vi "initialize.vi"(0 "HGF_FGV_Delete":refnum<class "HGF_FGV_Delete.lvclass">, 3 "initializationData":variant, 5 "error in (no error)":errorcluster, 7 "binaryString":string, 8 "I8 Array":i8[](array[numeric]), 9 "prependSize? (T)":bool, 11 "byteOrder (0:big-endian, network order)":T1(ring)) -> (14 "dup HGF_FGV_Delete":refnum<class "HGF_FGV_Delete.lvclass">, 17 "found?":bool, 19 "error out":errorcluster)   [LabVIEW 2012, in "HGF_FGV.lvlib" / "HGF_FGV_Delete.lvclass"]
doc: "This is a dynamic dispatch VI to be implemented by child classes to initialize their attributes.\n\n<B>Attention:</B> Support for Variant for initialization data only."
uses:
  HGF_FGV_Delete.lvclass
  HGF_FGV_Action/HGF_FGV_Action.lvclass
  HGF_FGV_Delete.lvclass/HGF_FGV_Delete.ctl
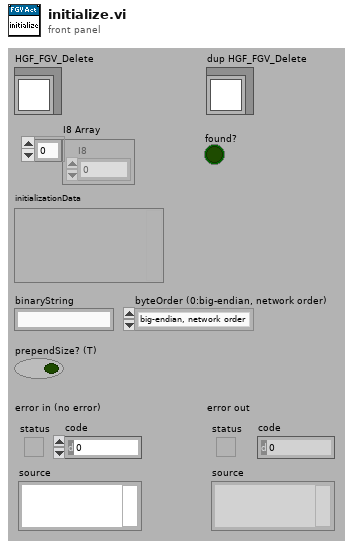
[diagram p1: front panel]
types:
  T1 = enum16{"big-endian, network order", "native, host order", "little-endian"}
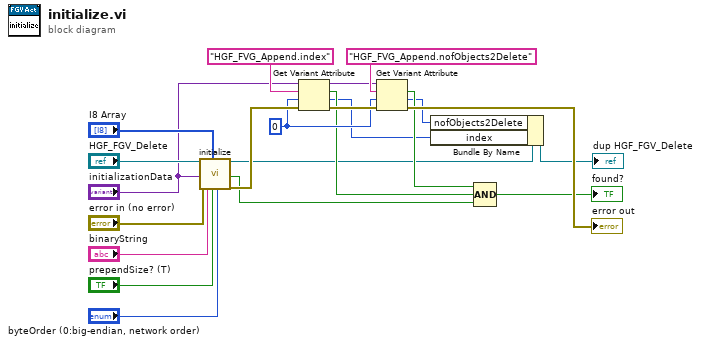
[diagram p0: block diagram]
diagram:
  w14 = u32 0
  n1 = call-parent "initialize.vi"("HGF_Factory"="HGF_FGV_Delete", "initializationData"="initializationData", "error in (no error)"="error in (no error)", "binaryString"="binaryString", "I8 Array"="I8 Array", "prependSize? (T)"="prependSize? (T)", "byteOrder (0:big-endian, network order)"="byteOrder (0:big-endian, network order)") -> ("dup HGF_Factory"=w7:refnum<class "HGF_FGV_Delete.lvclass">, "found?"=w16:bool, "error out"=w18:errorcluster)  [unwired: 1 in, 9 out]
  n2 = Get Variant Attribute(Variant="initializationData", name="HGF_FVG_Append.index", default value (empty Variant)=w14, error in=w18) -> (duplicate Variant=w10:variant, found=w9:bool, value=w5:u32, error out=w19:errorcluster)
  n3 = Get Variant Attribute(Variant=w10, name="HGF_FVG_Append.nofObjects2Delete", default value (empty Variant)=w14, error in=w19) -> (found=w8:bool, value=w6:u32, error out=→"error out":errorcluster)  [unwired: 1 out]
  n4 = Bundle By Name(cluster=w7, "nofObjects2Delete"=w6, "index"=w5) -> (→"dup HGF_FGV_Delete":refnum<class "HGF_FGV_Delete.lvclass">)
  n5 = Compound Arithmetic op=AND(w8, w9, w16) -> (→"found?":bool)
